vi "ContextHelpEditor VI.vi"(5 "Shift Pressed?":bool, 6 "ComboBox Text":string, 7 "Executed on Frontpanel?":bool, 8 "error in (no error)":errorcluster, 11 "VI Ref":refnum<vi>) -> (0 "error out":errorcluster)   [LabVIEW 2020, in "ContextHelpEditor.lvlib"]
uses:
  ContextHelpEditor.lvlib
  Data--cluster.ctl
  ControlRef--cluster.ctl
  <vilib>/picture/picture.llb/imagedata.ctl
  TabbedControl--cluster.ctl
  <vilib>/Platform/browser.llb/Open URL in Default Browser (string).vi
panel:
  in  "Controls":i32(listbox)
  in  "Help":bool
  in  "Delete VI Title":bool
  in  "VI Title":string caption="Title"
  in  "Description":string
  # "Use <b> and </b> tags around any text in the description you want to format as bold. \n\nUse TAB (forward) and SHIFT+TAB (backward) to jump between entries. \nESC will close the editor and change the VI properties. The VI won't be saved automatically."
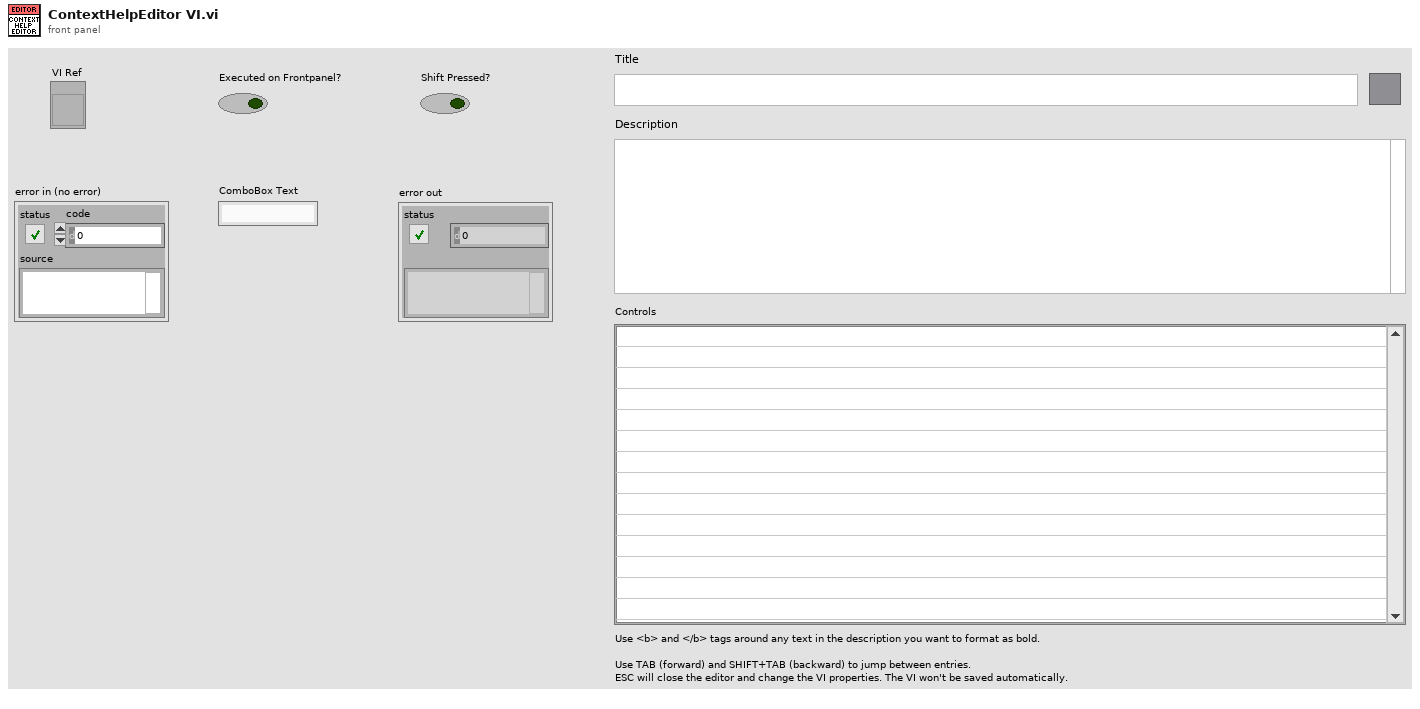
[diagram p1: front panel]
types:
  T1 = enum32{"Invalid", "Standard", "Closed", "Hidden", "Minimized", "Maximized"}
  T2 = enum32{"invalid app kind", "Development System", "Run Time System", "Student Edition", "Embedded LabVIEW", "Evaluation", "Custom"}
  T3 = typedef "ContextHelpEditor.lvlib/Data--cluster.ctl" = cluster{"Core":cluster{"Current VI Reference":refnum<vi>, "Close Panel on Exit?":bool}, "Controls":T4[], "QuickDrop":cluster{"VI Ref":refnum<vi>, "Executed on Frontpanel?":bool, "Shift Pressed?":bool, "ComboBox Text":string}, "TabbedControls":T6[]}
  T4 = typedef "ContextHelpEditor.lvlib/ControlRef--cluster.ctl" = cluster{"Ref":refnum<vi>, "Label":string, "Description":string, "Image":T5}
  T5 = typedef "imagedata.ctl" = cluster{"image type":i32, "image depth":i32, "image":u8[], "mask":u8[], "colors":u32[], "Rectangle":cluster{"left":i16, "top":i16, "right":i16, "bottom":i16}}
  T6 = typedef "ContextHelpEditor.lvlib/TabbedControl--cluster.ctl" = cluster{"Label":string, "Control Ref":refnum<vi>, "ClassName":string}
  T7 = enum32{"invalid VI type", "Standard VI", "Control VI", "Global VI", "Polymorphic VI", "Configuration VI", "SubSystem", "Facade VI", "Method VI", "Statechart Diagram VI"}
  T8 = typedef "eventvkey.ctl" = enum16{"ASCII", "Enter", "Return", "Shift", "Ctrl", "Alt", "Cmd", "Opt", "Caps", "NumLock", "Clear", "Break", "Up", "Down", "Left", "Right", "Insert", "Delete", "Home", "End", "PageUp", "PageDown", "Escape", "Help", "Pause", "ScrollLock", "F1", "F2", "F3", "F4", "F5", "F6", "F7", "F8", "F9", "F10", "F11", "F12", "F13", "F14", "F15", "F16", "F17", "F18", "F19", "F20", "F21", "F22", "F23", "F24", "Play", "VolumeUp", "VolumeDown", "Mute", "Two Byte Char"}
  T9 = cluster{"Shift":bool, "Ctrl":bool, "Alt":bool, "Cmd":bool, "Opt":bool}
  T10 = typedef "LVPoint32TypeDef.ctl" = cluster{"Horizontal":i32, "Vertical":i32}
  T11 = typedef "LVRowAndColumnTypeDef.ctl" = cluster{"Row":i32, "Column":i32}
  T12 = cluster{"Current VI Reference":refnum<vi>, "Close Panel on Exit?":bool}
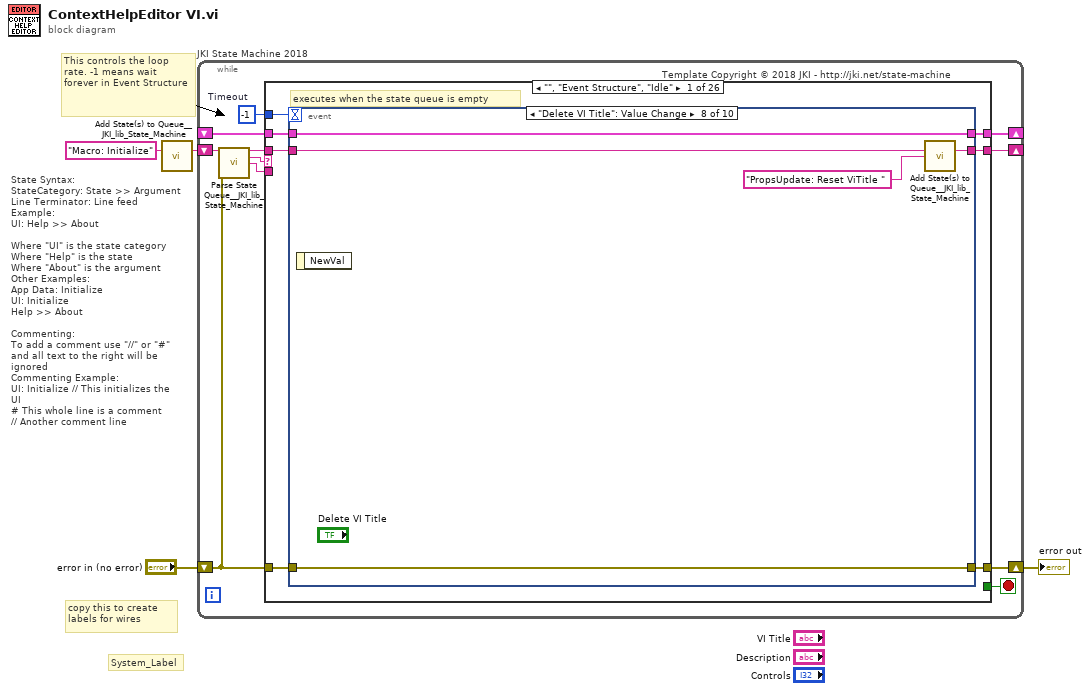
[diagram p0: block diagram]
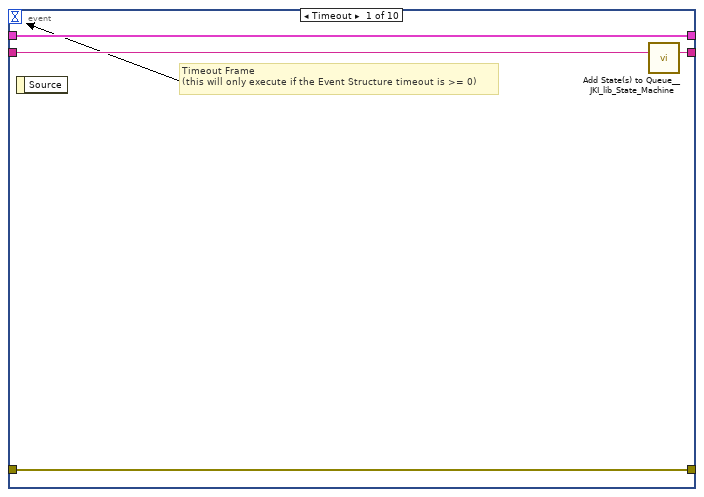
[diagram p2: hidden frame]
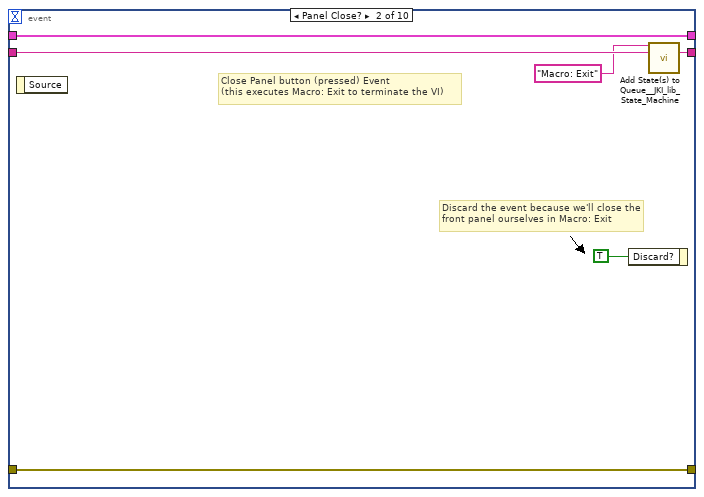
[diagram p3: hidden frame]
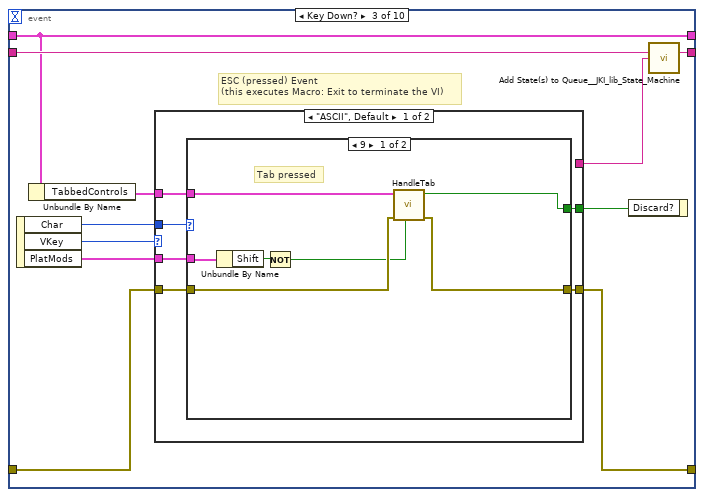
[diagram p4: hidden frame]
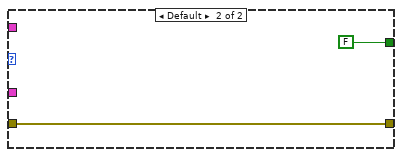
[diagram p5: hidden frame]
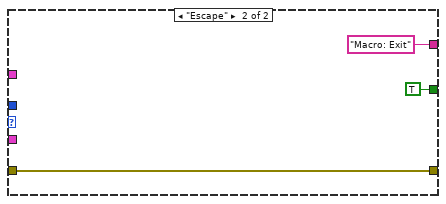
[diagram p6: hidden frame]
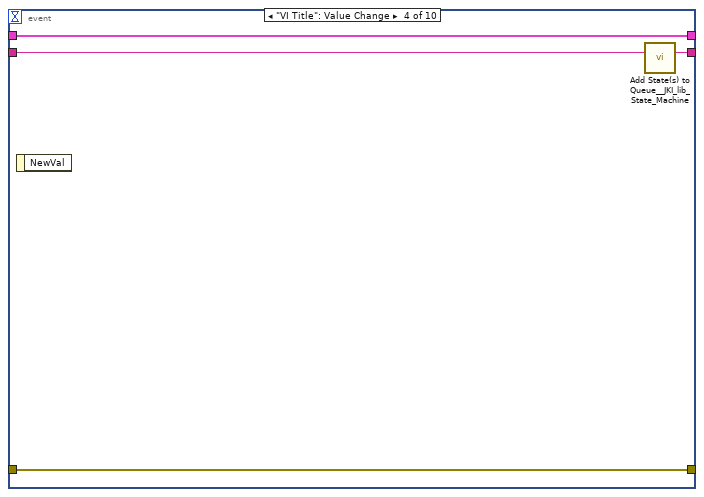
[diagram p7: hidden frame]
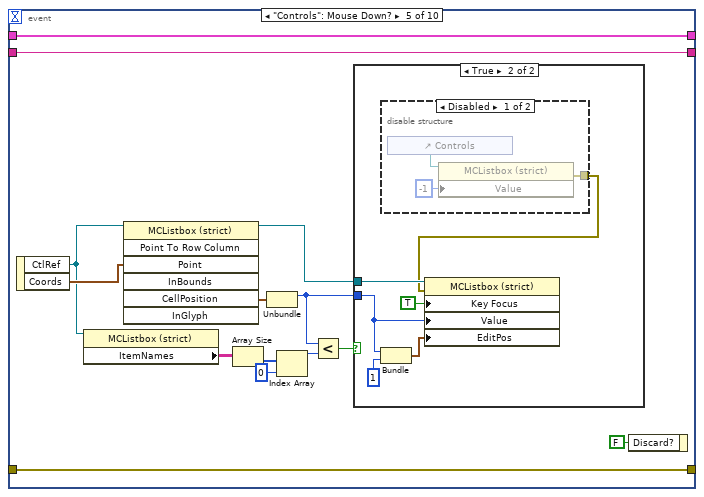
[diagram p8: hidden frame]
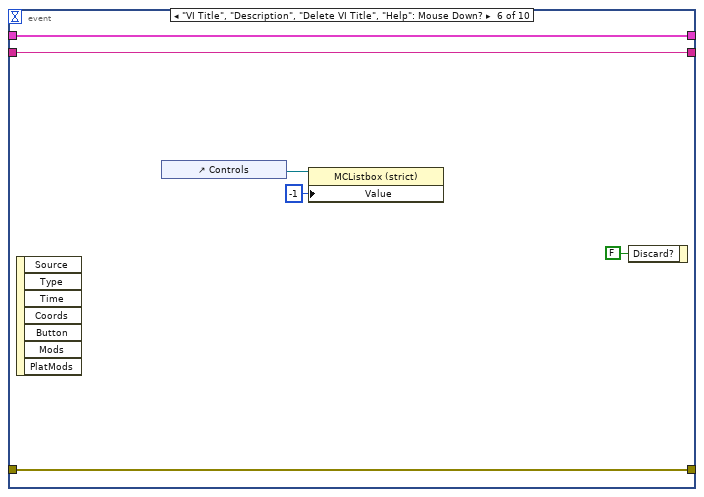
[diagram p11: hidden frame]
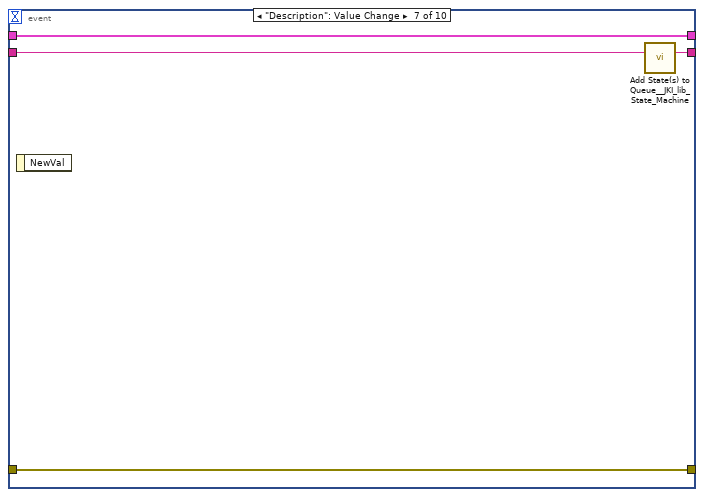
[diagram p12: hidden frame]
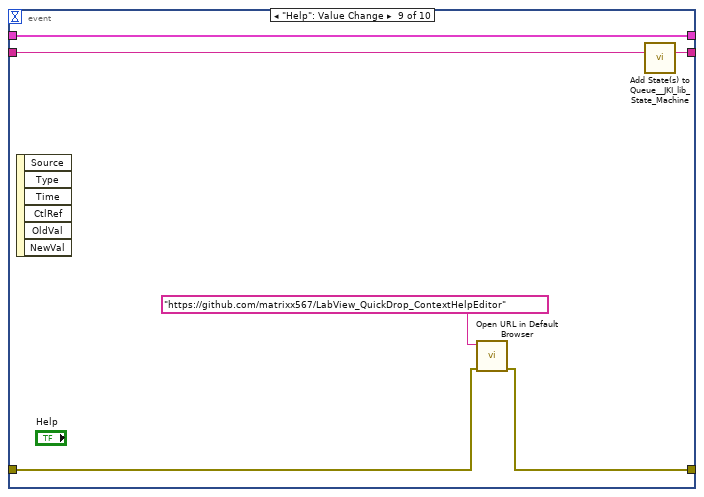
[diagram p13: hidden frame]
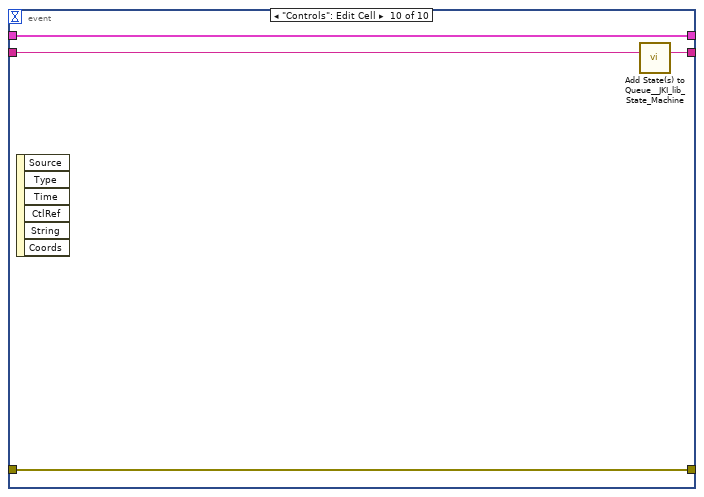
[diagram p14: hidden frame]
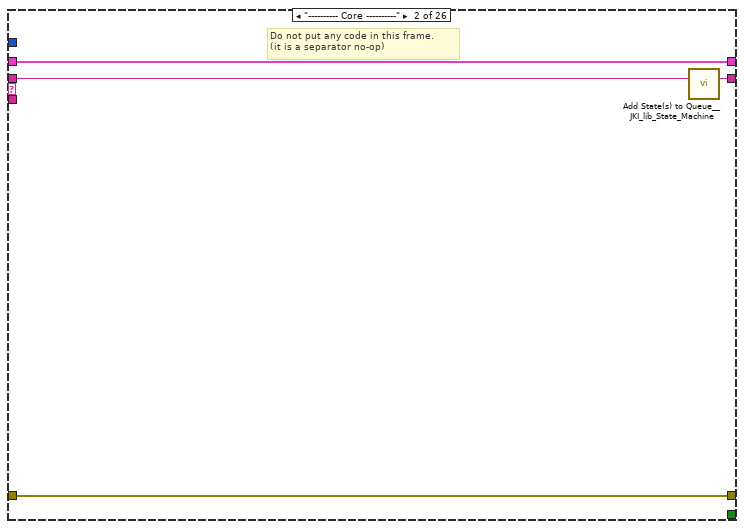
[diagram p15: hidden frame]
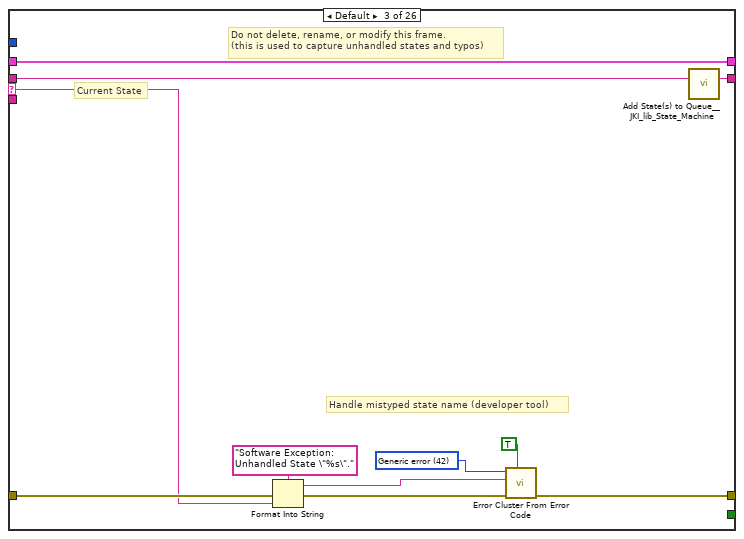
[diagram p16: hidden frame]
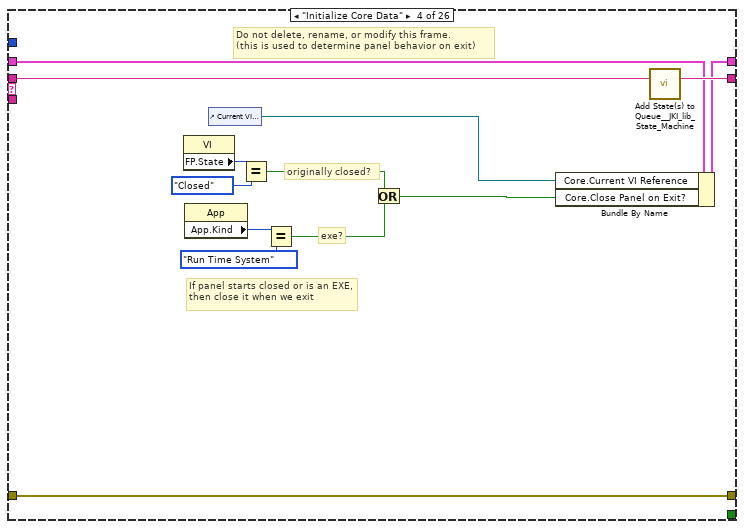
[diagram p17: hidden frame]
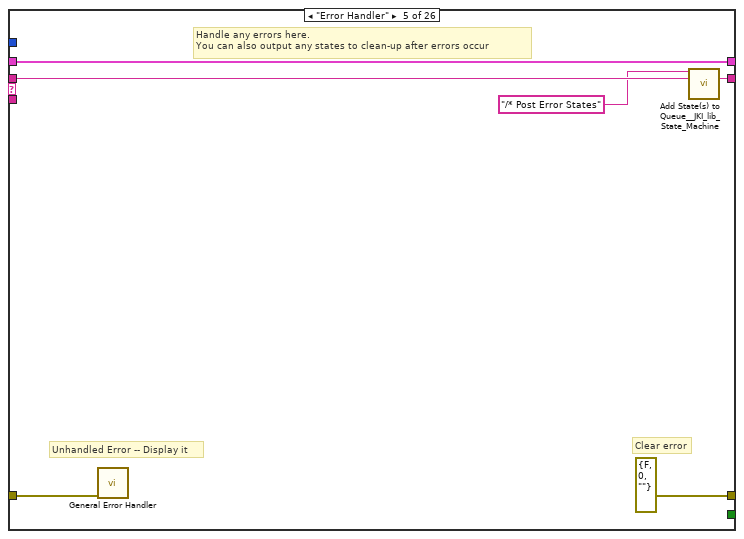
[diagram p18: hidden frame]
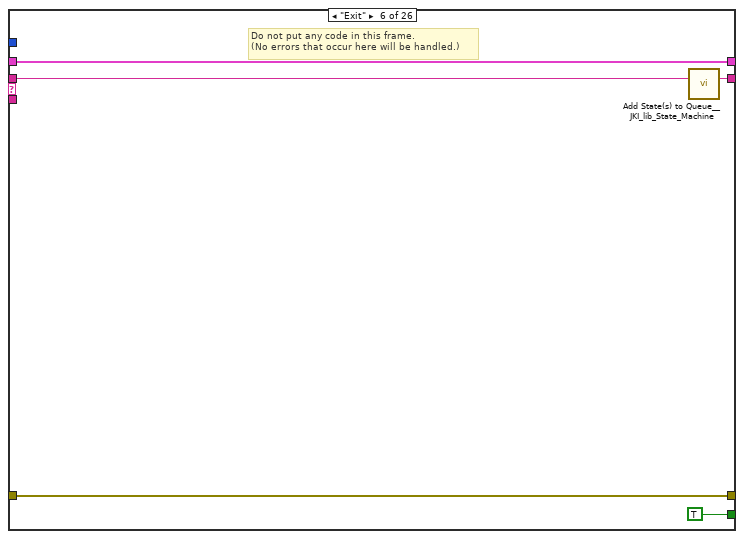
[diagram p19: hidden frame]
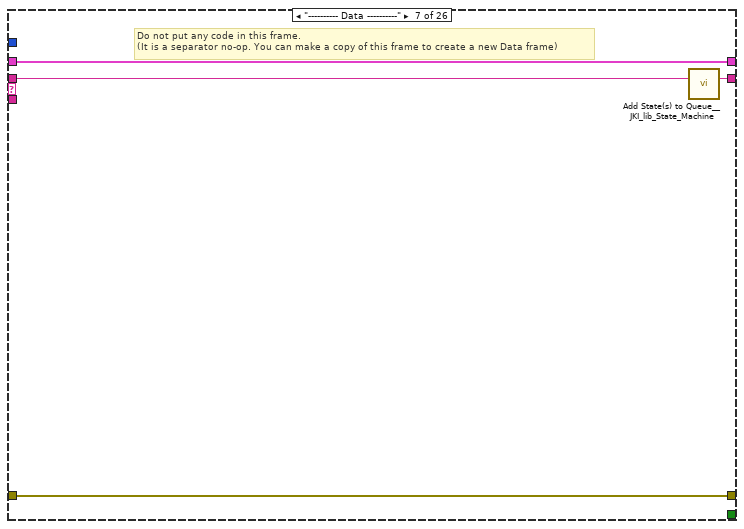
[diagram p20: hidden frame]
diagram:
  # "State Syntax:\nStateCategory: State >> Argument\nLine Terminator: Line feed\nExample:\nUI: Help >> About\n\nWhere \"UI\" is the state category\nWhere \"Help\" is the state\nWhere \"About\" is the argument\nOther Examples:\nApp Data: Initialize\nUI: Initialize\nHelp >> About\n\nCommenting:\nTo add a comment use \"//\" or \"#\" and all text to the right will be ignored\nCommenting Example:\nUI: Initialize // This initializes the UI\n# This whole line is a comment\n// Another comment line"
  # "copy this to create labels for wires"
  # "This controls the loop rate. -1 means wait forever in Event Structure"
  # "System_Label"
  n1 = call <vilib>:"Add State(s) to Queue__JKI_lib_State_Machine.vi"("State(s) in (\"\")"="Macro: Initialize") -> ("States Out"=w4:string)  [unwired: 14 in]
  n2 = while "JKI State Machine 2018" {
    shift-right: [w8] -> _
    shift-left: _ -> [w7]
    shift-right: [w11] -> w1
    shift-left: "error in (no error)" -> [w5]
    shift-right: [w10] -> _
    shift-left: w4 -> [w12]
    stop <- w9 stop-if-true
    w6 = -1  # Timeout
    # "Template Copyright © 2018 JKI - http://jki.net/state-machine"
    n3 = call <vilib>:"Parse State Queue__JKI_lib_State_Machine.vi"("State Queue"=w12, "Error In (no error)"=w5) -> ("Remaining States"=w14:string, "Current State"=w15:string, "Arguments"=w13:string)  [unwired: 11 in]
    n4 = case shown="\"\", \"Event Structure\", \"Idle\"" w15 {
      selector: w15 -> [_ _ w118 _ _ _ _ _ _ _ _ _ _ _ _ _ _ _ _ _ _ _ _ _ _ _]
      tunnel: w14 -> [w22 w117 w122 w141 w147 w152 w156 w167 w177 w194 w198 w210 w216 w227 w302 w314 w335 w354 w363 w368 w380 w384 w394 w406 w444 w478]
      tunnel: w13 -> [_ _ _ _ _ _ _ _ _ _ _ _ w211 w221 _ _ _ _ _ _ _ _ _ _ _ _]
      tunnel: w7 -> [w20 w114 w120 w134 w144 w150 w153 _ w174 w191 w195 w202 w214 w223 w295 w312 w333 w352 w360 w364 w377 w381 w391 w404 w442 w476]
      tunnel: [w19 w115 w124 w138 errorcluster {"status"=FALSE, "code"=0, "source"=""} ("error out") w149 w154 w162 w168 w190 w196 w201 w212 w224 w296 w310 w331 w351 w361 w366 w378 w382 w389 w396 w434 w473] -> w11
      tunnel: w5 -> [w18 w115 w123 w138 w143 w149 w154 w164 w170 w190 w196 w201 w213 w225 _ w309 _ _ w361 w366 w378 w382 w388 w395 w433 w472]
      tunnel: [w21 w116 w121 w140 w146 w151 w155 w166 w176 w193 w197 w209 w215 w226 w301 w313 w334 w353 w362 w367 w379 w383 w393 w405 w443 w477] -> w10
      tunnel: [_ _ _ _ _ TRUE _ _ _ _ _ _ _ _ _ _ _ _ _ _ _ _ _ _ _ _] -> w9
      tunnel: [w17 w114 w120 w139 w144 w150 w153 w165 w175 w191 w195 w202 w214 w223 w300 w312 w333 w352 w360 w364 w377 w381 w391 w404 w442 w476] -> w8
      tunnel: w6 -> [w16 _ _ _ _ _ _ _ _ _ _ _ _ _ _ _ _ _ _ _ _ _ _ _ _ _]
      frame "", "Event Structure", "Idle" {
        # "executes when the state queue is empty"
        n5 = event shown="[7] \"Delete VI Title\": Value Change" {
          selector: _ -> [_ _ _ _ _ _ _ _ _ _]
          dyn-events: _ -> [_ _ _ _ _ _ _ _ _ _]
          timeout: w16 -> [_ _ _ _ _ _ _ _ _ _]
          tunnel: w22 -> [w26 w32 w43 w64 w79 w94 w97 w102 w108 w112]
          tunnel: [w25 w31 w42 w65 w79 w94 w98 w103 w109 w111] -> w21
          tunnel: w20 -> [w23 w29 w36 w63 w77 w92 w96 w101 w107 w113]
          tunnel: [w24 w30 w37 w62 w78 w93 w95 w99 w104 w110] -> w19
          tunnel: w18 -> [w24 w30 w38 w62 w78 w93 w95 w99 w105 w110]
          tunnel: [w23 w29 w36 w63 w77 w92 w96 w101 w107 w113] -> w17
          event Timeout {
            # "Timeout Frame\n(this will only execute if the Event Structure timeout is >= 0)"
            n6 = event-data() -> ()  [unwired: 1 in, 1 out]
            n7 = call <vilib>:"Add State(s) to Queue__JKI_lib_State_Machine.vi"("State(s) in (\"\")"=w26) -> ("States Out"=w25:string)  [unwired: 14 in]
          }
          event Panel Close? {
            # "Discard the event because we'll close the front panel ourselves in Macro: Exit"
            # "Close Panel button (pressed) Event\n(this executes Macro: Exit to terminate the VI)"
            n8 = event-data() -> ()  [unwired: 1 in, 1 out]
            n9 = event-data("Discard?"=TRUE) -> ()  [unwired: 1 in, 1 out]
            n10 = call <vilib>:"Add State(s) to Queue__JKI_lib_State_Machine.vi"("State(s) in Front (\"\")"="Macro: Exit", "State(s) in (\"\")"=w32) -> ("States Out"=w31:string)  [unwired: 13 in]
          }
          event Key Down? {
            # "ESC (pressed) Event\n(this executes Macro: Exit to terminate the VI)"
            n11 = event-data() -> ("Char"=w39:i16, "VKey"=w41:T8, "PlatMods"=w34:T9)  [unwired: 1 in]
            n12 = Unbundle By Name(w36) -> ("TabbedControls"=w35:T6[])
            n13 = case shown="\"ASCII\", Default" w41 {
              tunnel: [_ "Macro: Exit"] -> w33
              tunnel: [w48 TRUE] -> w40
              tunnel: w39 -> [w49 _]
              tunnel: [w47 w61] -> w37
              tunnel: w38 -> [w46 w61]
              tunnel: w35 -> [w45 _]
              tunnel: w34 -> [w44 _]
              frame "ASCII", Default {
                n14 = case shown="9" w49 {
                  tunnel: [w56 FALSE] -> w48
                  tunnel: [w54 w57] -> w47
                  tunnel: w46 -> [w55 w57]
                  tunnel: w45 -> [w53 _]
                  tunnel: w44 -> [w52 _]
                  frame 9 {
                    # "Tab pressed"
                    n15 = Unbundle By Name(w52) -> ("Shift"=w51:bool)
                    n16 = Not(x=w51) -> (.not. x?=w50:bool)
                    n17 = call "HandleTab.vi"("Forward?"=w50, "error in (no error)"=w55, "TabbedControls"=w53) -> ("error out"=w54:errorcluster, "Discard?"=w56:bool)  [unwired: 7 in]
                  }
                  frame Default {
                  }
                }
              }
              frame "Escape" {
              }
            }
            n18 = event-data("Discard?"=w40) -> ()  [unwired: 1 in, 1 out]
            n19 = call <vilib>:"Add State(s) to Queue__JKI_lib_State_Machine.vi"("State(s) in (\"\")"=w43, "State(s) at Back (\"\")"=w33) -> ("States Out"=w42:string)  [unwired: 13 in]
          }
          event "VI Title": Value Change {
            n20 = event-data() -> ()  [unwired: 1 in, 1 out]
            n21 = call <vilib>:"Add State(s) to Queue__JKI_lib_State_Machine.vi"("State(s) in (\"\")"=w64) -> ("States Out"=w65:string)  [unwired: 14 in]
          }
          event "Controls": Mouse Down? {
            n22 = event-data() -> ("CtlRef"=w72:refnum<vi>, "Coords"=w76:T10)  [unwired: 1 in]
            n23 = property class="MCListbox (strict)"(reference=w72) -> ("ItemNames"=w71:string[][])  [unwired: 1 in, 2 out]
            n24 = invoke class="MCListbox (strict)" method="Point To Row Column"(reference=w72, "Point"=w76) -> (reference out=w75:refnum<vi>, "CellPosition"=w74:T11)  [unwired: 5 in, 5 out]
            n25 = Array Size(array=w71) -> (size(s)=w67:i32[])
            n26 = Unbundle(w74) -> ("Row"=w70:i32)  [unwired: 1 out]
            n27 = Index Array(array=w67, index=0) -> (element=w66:i32)
            n28 = Less?(x=w70, y=w66) -> (x < y?=w69:bool)
            n29 = case shown="True" w69 {
              tunnel: w75 -> [_ w83]
              tunnel: w70 -> [_ w80]
              frame False {
                # "ignore empty lines"
              }
              frame True {
                n30 = Bundle("Row"=w80, "Row"=1) -> (w85:cluster{"Row":i32, "Row":i32})  [unwired: 1 in]
                n31 = disable-structure shown="Disabled" {
                  disable-tunnel: [w87 _] -> w81
                  frame Disabled {
                    n32 = control-ref of="Controls"() -> (w88:refnum<vi>)
                    n33 = property class="MCListbox (strict)"(reference=w88, "Value"=-1) -> (error out=w87:errorcluster)  [unwired: 1 in, 1 out]
                  }
                  frame Enabled {
                  }
                }
                n34 = property class="MCListbox (strict)"(reference=w83, error in=w81, "Key Focus"=TRUE, "Value"=w80, "EditPos"=w85) -> ()  [unwired: 2 out]
              }
            }
            n35 = event-data("Discard?"=FALSE) -> ()  [unwired: 1 in, 1 out]
          }
          event "VI Title", "Description", "Delete VI Title", "Help": Mouse Down? {
            n36 = event-data() -> ()  [unwired: 1 in, 7 out]
            n37 = control-ref of="Controls"() -> (w90:refnum<vi>)
            n38 = property class="MCListbox (strict)"(reference=w90, "Value"=-1) -> ()  [unwired: 1 in, 2 out]
            n39 = event-data("Discard?"=FALSE) -> ()  [unwired: 1 in, 1 out]
          }
          event "Description": Value Change {
            n40 = event-data() -> ()  [unwired: 1 in, 1 out]
            n41 = call <vilib>:"Add State(s) to Queue__JKI_lib_State_Machine.vi"("State(s) in (\"\")"=w97) -> ("States Out"=w98:string)  [unwired: 14 in]
          }
          event "Delete VI Title": Value Change {
            n42 = event-data() -> ()  [unwired: 1 in, 1 out]
            n43 = call <vilib>:"Add State(s) to Queue__JKI_lib_State_Machine.vi"("State(s) in (\"\")"=w102, "State(s) at Back (\"\")"="PropsUpdate: Reset ViTitle ") -> ("States Out"=w103:string)  [unwired: 13 in]
          }
          event "Help": Value Change {
            n44 = event-data() -> ()  [unwired: 1 in, 6 out]
            n45 = call-poly <vilib>:"Open URL in Default Browser.vi"("error in (no error)"=w105, "URL"="https://github.com/matrixx567/LabView_QuickDrop_ContextHelpEditor") -> ("error out"=w104:errorcluster)  [unwired: 4 in, 1 out]
            n46 = call <vilib>:"Add State(s) to Queue__JKI_lib_State_Machine.vi"("State(s) in (\"\")"=w108) -> ("States Out"=w109:string)  [unwired: 14 in]
          }
          event "Controls": Edit Cell {
            n47 = event-data() -> ()  [unwired: 1 in, 6 out]
            n48 = call <vilib>:"Add State(s) to Queue__JKI_lib_State_Machine.vi"("State(s) in (\"\")"=w112) -> ("States Out"=w111:string)  [unwired: 14 in]
          }
        }
      }
      frame "---------- Core ----------" {
        # "Do not put any code in this frame.\n(it is a separator no-op)"
        n49 = call <vilib>:"Add State(s) to Queue__JKI_lib_State_Machine.vi"("State(s) in (\"\")"=w117) -> ("States Out"=w116:string)  [unwired: 14 in]
      }
      frame Default {
        w127 = 42 items=["No error", "Argument error", "Memory is full", "Out of zone", "End of file", "File already open", "Generic file I/O error", "File not found", "File permission error", "Disk is full", "Duplicate path", "Too many files open", "System feature not enabled", "Resource file not found", "Cannot add resource", "Resource not found", "Image not found", "Image memory error", "Pen does not exist", "Config type invalid", "Config token not found", "Config parse error", "Config memory error", "Bad external code format", "Bad external code offset", "External code not present", "Null window", "Destroy window error", "Null menu", "Print aborted", "Bad print record", "Print driver error", "Windows error during printing", "Memory error during printing", "Print dialog error", "Generic print error", "Invalid device refnum", "Device not found", "Device parameter error", "Device unit error", "Cannot open device", "Device call aborted", "Generic error", "Cancelled by user", "Object ID too low", "Object ID too high", "Object not in heap", "Unknown heap", "Unknown object (invalid DefProc)", "Unknown object (DefProc not in table)", "Message out of range", "Invalid (null) method", "Unknown message", "Manager call not supported", "Bad address", "Network operation in progress", "Network operation timed out", "Connection is busy", "Network attribute not supported", "Network error", "Address in use", "System out of memory", "Connection aborted", "Connection refused", "Not connected", "Already connected", "Connection closed", "Initialization error (interapplication manager)", "Bad occurrence", "Wait on unbound occurrence handler", "Occurrence queue overflow", "Datalog type conflict", "Unused", "Unrecognized type (interapplication manager)", "Memory corrupt", "Failed to make temporary DLL", "Old CIN version", "Drag socket not found", "Failed to load drop-object", "Failed to register OLE object", "Failed to release OLE object", "Format specifier type mismatch", "Unknown format specifier", "Too few format specifiers", "Too many format specifiers", "Scan failed", "Newer CIN version", "Error converting to variant", "Runtime menu error", "Password tampered", "Variant attribute not found", "Incompatible variant data type", "Event data is not available", "Event Store is not present", "Occurrence is not found", "Event Queue is not created", "Event info is not available", "Refnum passed is NULL", "Error retrieving Class GUID", "Error retrieving CoClass GUID", "Error retrieving TypeLib GUID.", "Bad built application magic bytes.", "Specific driver is different from the specific driver associated with the Logical Name.", "There is no session opened to the class driver.", "Max Error", "MAX - Error with config objects", "MAX - Error loading configuration", "MAX - Group not supported"]
        # "Current State"
        # "Do not delete, rename, or modify this frame.\n(this is used to capture unhandled states and typos)"
        # "Handle mistyped state name (developer tool)"
        n50 = Format Into String(format string="Software Exception: Unhandled State \"%s\"." ("message"), error in=w123, w118) -> (resulting string=w126:string, error out=w125:errorcluster)  [unwired: 1 in]
        n51 = call <vilib>:"Error Cluster From Error Code.vi"("show call chain? (False)"=TRUE, "error in (no error)"=w125, "error message (\"\")"=w126, "error code (0)"=w127) -> ("error out"=w124:errorcluster)  [unwired: 5 in]
        n52 = call <vilib>:"Add State(s) to Queue__JKI_lib_State_Machine.vi"("State(s) in (\"\")"=w122) -> ("States Out"=w121:string)  [unwired: 14 in]
      }
      frame "Initialize Core Data" {
        # "Do not delete, rename, or modify this frame.\n(this is used to determine panel behavior on exit)"
        # "originally closed?"
        # "exe?"
        # "If panel starts closed or is an EXE, then close it when we exit"
        n53 = property class="VI"() -> ("FP.State"=w131:T1)  [unwired: 2 in, 2 out]
        n54 = property class="App"() -> ("App.Kind"=w137:T2)  [unwired: 2 in, 2 out]
        n55 = control-ref of="Current VI Reference"() -> (w132:refnum<vi>)
        n56 = Equal?(x=w131, y=T1."Closed" ("Front Panel Window:State")) -> (x = y?=w129:bool)
        n57 = Equal?(x=w137, y=T2."Run Time System" ("Application:Kind")) -> (x = y?=w135:bool)
        n58 = Or(x=w129, y=w135) -> (x .or. y?=w133:bool)
        n59 = Bundle By Name(cluster=w134, "Core.Current VI Reference"=w132, "Core.Close Panel on Exit?"=w133) -> (w139:T3)
        n60 = call <vilib>:"Add State(s) to Queue__JKI_lib_State_Machine.vi"("State(s) in (\"\")"=w141) -> ("States Out"=w140:string)  [unwired: 14 in]
      }
      frame "Error Handler" {
        # "Unhandled Error -- Display it"
        # "Handle any errors here.\nYou can also output any states to clean-up after errors occur"
        # "Clear error"
        n61 = call <vilib>:"General Error Handler.vi"("error in (no error)"=w143) -> ()  [unwired: 10 in, 5 out]
        n62 = call <vilib>:"Add State(s) to Queue__JKI_lib_State_Machine.vi"("State(s) in Front (\"\")"="/* Post Error States", "State(s) in (\"\")"=w147) -> ("States Out"=w146:string)  [unwired: 13 in]
      }
      frame "Exit" {
        # "Do not put any code in this frame.\n(No errors that occur here will be handled.)"
        n63 = call <vilib>:"Add State(s) to Queue__JKI_lib_State_Machine.vi"("State(s) in (\"\")"=w152) -> ("States Out"=w151:string)  [unwired: 14 in]
      }
      frame "---------- Data ----------" {
        # "Do not put any code in this frame.\n(It is a separator no-op. You can make a copy of this frame to create a new Data frame)"
        n64 = call <vilib>:"Add State(s) to Queue__JKI_lib_State_Machine.vi"("State(s) in (\"\")"=w156) -> ("States Out"=w155:string)  [unwired: 14 in]
      }
      frame "Data: Initialize" {
        w163 = T12 {"Current VI Reference"=refnum, "Close Panel on Exit?"=FALSE}  # Core
        # "do not delete - used by framework"
        # "Data names and types of shift register data are defined by this bundle."
        # "Initialize the shift-register data, here.\n(data names are defined by what you wire into the bundle function)"
        n65 = Merge Errors(w164) -> (w162:errorcluster)
        n66 = Bundle By Name(cluster=T3 {"Core"={"Current VI Reference"=refnum, "Close Panel on Exit?"=FALSE}, "Controls"=[], "QuickDrop"={"VI Ref"=refnum, "Executed on Frontpanel?"=FALSE, "Shift Pressed?"=FALSE, "ComboBox Text"=""}, "TabbedControls"=[]}, "Core"=w163, "QuickDrop.VI Ref"="VI Ref", "QuickDrop.Executed on Frontpanel?"="Executed on Frontpanel?", "QuickDrop.ComboBox Text"="ComboBox Text", "QuickDrop.Shift Pressed?"="Shift Pressed?") -> (w165:T3)
        n67 = call <vilib>:"Add State(s) to Queue__JKI_lib_State_Machine.vi"("State(s) in (\"\")"=w167) -> ("States Out"=w166:string)  [unwired: 14 in]
      }
      frame "Data: LoadControlFromVI" {
        # "Initialize the shift-register data, here.\n(data names are defined by what you wire into the bundle function)"
        n68 = Unbundle By Name(w174) -> ("QuickDrop.VI Ref"=w172:refnum<vi>)
        n69 = property class="VI"(reference=w172) -> ("VIType"=w171:T7)  [unwired: 1 in, 2 out]
        n70 = case shown="\"Control VI\"" w171 {
          tunnel: w172 -> [_ w181 w189]
          tunnel: [_ w180 w187] -> w173
          tunnel: [_ w178 w188] -> w169
          frame Default {
          }
          frame "Standard VI" {
            w182 = FALSE  # LoadAllControls
            n71 = call "ExtractControlRefsFromVi.vi"("ShowAllControls?"=w182, "VI in"=w181) -> ("error out"=w186:errorcluster, "Controls"=w183:T4[])  [unwired: 8 in]
            n72 = call "ExtractControlRefsFromVi.vi"("Indicators"=TRUE, "ShowAllControls?"=w182, "VI in"=w181) -> ("error out"=w185:errorcluster, "Controls"=w179:T4[])  [unwired: 7 in]
            n73 = Merge Errors(w186, w185) -> (w178:errorcluster)
            n74 = Build Array (concatenate)(w183, w179) -> (w180:T4[])
          }
          frame "Control VI" {
            n75 = call "ExtractControlRefsFromTypedef.vi"("VI in"=w189) -> ("error out"=w188:errorcluster, "Controls"=w187:T4[])  [unwired: 9 in]
          }
        }
        n76 = Bundle By Name(cluster=w174, "Controls"=w173) -> (w175:T3)
        n77 = Merge Errors(w170, w169) -> (w168:errorcluster)
        n78 = call <vilib>:"Add State(s) to Queue__JKI_lib_State_Machine.vi"("State(s) in (\"\")"=w177) -> ("States Out"=w176:string)  [unwired: 14 in]
      }
      frame "Data: Cleanup" {
        # "Cleanup any data and references, here.\n(this is called automatically, by the Macro: Exit)"
        n79 = Unbundle By Name(w191) -> ("Core.Current VI Reference"=w192:refnum<vi>)
        n80 = Close Reference(reference=w192) -> ()  [unwired: 1 in, 1 out]
        n81 = call <vilib>:"Add State(s) to Queue__JKI_lib_State_Machine.vi"("State(s) in (\"\")"=w194) -> ("States Out"=w193:string)  [unwired: 14 in]
      }
      frame "---------- UI ----------" {
        # "Do not put any code in this frame.\n(It is a separator no-op. You can make a copy of this frame to create a new UI frame)"
        n82 = call <vilib>:"Add State(s) to Queue__JKI_lib_State_Machine.vi"("State(s) in (\"\")"=w198) -> ("States Out"=w197:string)  [unwired: 14 in]
      }
      frame "UI: Initialize" {
        # "Initialize the User Interface, here.\n(this is called automatically, by the Macro: Init)"
        n83 = Unbundle By Name(w202) -> ("Core.Current VI Reference"=w207:refnum<vi>)
        n84 = Unbundle By Name(w202) -> ("QuickDrop.VI Ref"=w204:refnum<vi>)
        n85 = property class="VI"(reference=w204) -> ("Front Panel.Title"=w203:string)  [unwired: 1 in, 2 out]
        n86 = control-ref of="Controls"() -> (w208:refnum<vi>)
        n87 = Concatenate Strings("ContextHelpEditor - " ("string"), w203) -> (w206:string)
        n88 = property class="VI"(reference=w207, "Front Panel.Title"=w206) -> ()  [unwired: 1 in, 2 out]
        n89 = property class="MCListbox (strict)"(reference=w208, "SelColor"=u32 13816530, "Value"=-1) -> ()  [unwired: 1 in, 2 out]
        n90 = call <vilib>:"Add State(s) to Queue__JKI_lib_State_Machine.vi"("State(s) in (\"\")"=w210) -> ("States Out"=w209:string)  [unwired: 14 in]
      }
      frame "UI: Cursor Set" {
        # "Argument"
        # "Set and Unset Cursor Busy.\n(Usage: \"UI: Cursor Set >> Busy|Idle\")"
        n91 = case shown="\"Busy\"" w211 {
          tunnel: w213 -> [w218 w220]
          tunnel: [w217 w219] -> w212
          frame "Idle", Default {
            n92 = call <vilib>:"Unset Busy.vi"("error in (no error)"=w218) -> ("error out"=w217:errorcluster)  [unwired: 10 in]
          }
          frame "Busy" {
            n93 = call <vilib>:"Set Busy.vi"("error in (no error)"=w220) -> ("error out"=w219:errorcluster)  [unwired: 9 in, 1 out]
          }
        }
        n94 = call <vilib>:"Add State(s) to Queue__JKI_lib_State_Machine.vi"("State(s) in (\"\")"=w216) -> ("States Out"=w215:string)  [unwired: 14 in]
      }
      frame "UI: Front Panel State" {
        # "Argument"
        # "Set Front Panel Open or Closed\n(Usage: \"UI: Front Panel State >> Open|Close\")"
        n95 = Unbundle By Name(w223) -> ("Core.Current VI Reference"=w222:refnum<vi>)
        n96 = case shown="\"Open\", \"Standard\", Default" w221 {
          tunnel: w225 -> [w233 w248 w259 w272 w285]
          tunnel: [w235 w249 w261 w274 w287] -> w224
          tunnel: w222 -> [w234 w246 w260 w273 w286]
          frame "Open", "Standard", Default {
            w228 = T1."Standard" ("State")
            n97 = property class="VI"(reference=w234, error in=w233) -> (reference out=w231:refnum<vi>, error out=w232:errorcluster, "FP.State"=w230:T1)
            n98 = Not Equal?(x=w230, y=w228) -> (x != y?=w229:bool)
            n99 = case shown="True" w229 {
              tunnel: [w239 w241] -> w235
              tunnel: w232 -> [w238 w241]
              tunnel: w231 -> [w237 _]
              tunnel: w228 -> [w236 _]
              frame True {
                n100 = invoke class="VI" method="FP.Open"(reference=w237, error in=w238, "Activate"=TRUE, "State"=w236) -> (error out=w239:errorcluster)  [unwired: 1 in, 4 out]
              }
              frame False {
              }
            }
          }
          frame "Close", "Closed" {
            n101 = property class="VI"(reference=w246, error in=w248) -> (reference out=w245:refnum<vi>, error out=w247:errorcluster, "FP.State"=w243:T1)
            n102 = Not Equal?(x=w243, y=T1."Closed" ("Front Panel Window:State")) -> (x != y?=w242:bool)
            n103 = case shown="True" w242 {
              tunnel: [w250 w253] -> w249
              tunnel: w247 -> [w250 w252]
              tunnel: w245 -> [_ w251]
              frame False {
              }
              frame True {
                n104 = invoke class="VI" method="FP.Close"(reference=w251, error in=w252) -> (error out=w253:errorcluster)  [unwired: 1 in, 2 out]
              }
            }
          }
          frame "Hidden", "Hide" {
            w254 = T1."Hidden" ("State")
            n105 = property class="VI"(reference=w260, error in=w259) -> (reference out=w257:refnum<vi>, error out=w258:errorcluster, "FP.State"=w256:T1)
            n106 = Not Equal?(x=w256, y=w254) -> (x != y?=w255:bool)
            n107 = case shown="True" w255 {
              tunnel: [w265 w266] -> w261
              tunnel: w258 -> [w264 w266]
              tunnel: w257 -> [w263 _]
              tunnel: w254 -> [w262 _]
              frame True {
                n108 = invoke class="VI" method="FP.Open"(reference=w263, error in=w264, "State"=w262) -> (error out=w265:errorcluster)  [unwired: 2 in, 4 out]
              }
              frame False {
              }
            }
          }
          frame "Minimize", "Minimized" {
            w267 = T1."Minimized" ("State")
            n109 = property class="VI"(reference=w273, error in=w272) -> (reference out=w270:refnum<vi>, error out=w271:errorcluster, "FP.State"=w269:T1)
            n110 = Not Equal?(x=w269, y=w267) -> (x != y?=w268:bool)
            n111 = case shown="True" w268 {
              tunnel: [w278 w279] -> w274
              tunnel: w271 -> [w277 w279]
              tunnel: w270 -> [w276 _]
              tunnel: w267 -> [w275 _]
              frame True {
                n112 = invoke class="VI" method="FP.Open"(reference=w276, error in=w277, "State"=w275) -> (error out=w278:errorcluster)  [unwired: 2 in, 4 out]
              }
              frame False {
              }
            }
          }
          frame "Maximize", "Maximized" {
            w280 = T1."Maximized" ("State")
            n113 = property class="VI"(reference=w286, error in=w285) -> (reference out=w283:refnum<vi>, error out=w284:errorcluster, "FP.State"=w282:T1)
            n114 = Not Equal?(x=w282, y=w280) -> (x != y?=w281:bool)
            n115 = case shown="True" w281 {
              tunnel: [w291 w292] -> w287
              tunnel: w284 -> [w290 w292]
              tunnel: w283 -> [w289 _]
              tunnel: w280 -> [w288 _]
              frame True {
                n116 = invoke class="VI" method="FP.Open"(reference=w289, error in=w290, "State"=w288) -> (error out=w291:errorcluster)  [unwired: 2 in, 4 out]
              }
              frame False {
              }
            }
          }
        }
        n117 = call <vilib>:"Add State(s) to Queue__JKI_lib_State_Machine.vi"("State(s) in (\"\")"=w227) -> ("States Out"=w226:string)  [unwired: 14 in]
      }
      frame "UI: LoadTabbedControls" {
        # "Initialize the User Interface, here.\n(this is called automatically, by the Macro: Init)"
        n118 = Unbundle By Name(w295) -> ("Core.Current VI Reference"=w299:refnum<vi>)
        n119 = control-ref of="Controls"() -> (w297:refnum<vi>)
        n120 = call "LoadTabbedControls.vi"("VI in"=w299) -> ("error out"=w296:errorcluster, "TabbedControls"=w298:T6[])  [unwired: 9 in]
        n121 = Bundle By Name(cluster=w295, "TabbedControls"=w298) -> (w300:T3)
        n122 = property class="MCListbox (strict)"(reference=w297, "SelColor"=u32 13816530, "Value"=-1) -> ()  [unwired: 1 in, 2 out]
        n123 = call <vilib>:"Add State(s) to Queue__JKI_lib_State_Machine.vi"("State(s) in (\"\")"=w302) -> ("States Out"=w301:string)  [unwired: 14 in]
      }
      frame "UI: VI Title String Update" {
        # "Do not put any code in this frame.\n(It is a separator no-op. You can make a copy of this frame to create a new UI frame)"
        n124 = Unbundle By Name(w312) -> ("Controls"=w303:T4[], "QuickDrop.VI Ref"=w305:refnum<vi>)
        n125 = property class="VI"(reference=w305) -> ("VIType"=w307:T7)  [unwired: 1 in, 2 out]
        n126 = Equal?(x=w307, y=T7."Control VI") -> (x = y?=w304:bool)
        n127 = case shown="False" w304 {
          tunnel: [w320 w321] -> w311
          tunnel: [w316 w322] -> w308
          tunnel: w305 -> [w315 _]
          tunnel: w303 -> [_ w325]
          frame False {
            n128 = property class="VI"(reference=w315) -> (error out=w320:errorcluster, "Front Panel.Title"=w318:string, "Front Panel.CustomTitle"=w319:bool, "Name"=w317:string)  [unwired: 1 in, 1 out]
            n129 = Select(t=w318, s=w319, f=w317) -> (s? t:f=w316:string)
          }
          frame True {
            n130 = Index Array(array=w325) -> (element=w324:T4)  [unwired: 1 in]
            n131 = Unbundle By Name(w324) -> ("Ref"=w323:refnum<vi>)
            n132 = property class="Ctl"(reference=w323) -> (error out=w321:errorcluster, "Label.Text"=w322:string)  [unwired: 1 in, 1 out]
          }
        }
        n133 = local write "VI Title"(w308) -> ()
        n134 = Merge Errors(w309, w311) -> (w310:errorcluster)
        n135 = call <vilib>:"Add State(s) to Queue__JKI_lib_State_Machine.vi"("State(s) in (\"\")"=w314) -> ("States Out"=w313:string)  [unwired: 14 in]
      }
      frame "UI: VI Description String Update" {
        # "Do not put any code in this frame.\n(It is a separator no-op. You can make a copy of this frame to create a new UI frame)"
        n136 = Unbundle By Name(w333) -> ("Controls"=w326:T4[], "QuickDrop.VI Ref"=w328:refnum<vi>)
        n137 = property class="VI"(reference=w328) -> ("VIType"=w330:T7)  [unwired: 1 in, 2 out]
        n138 = Equal?(x=w330, y=T7."Control VI") -> (x = y?=w327:bool)
        n139 = case shown="True" w327 {
          tunnel: [w338 w339] -> w332
          tunnel: [w337 w341] -> w331
          tunnel: w328 -> [w336 _]
          tunnel: w326 -> [_ w343]
          frame False {
            n140 = property class="VI"(reference=w336) -> (error out=w337:errorcluster, "Description"=w338:string)  [unwired: 1 in, 1 out]
          }
          frame True {
            n141 = Index Array(array=w343) -> (element=w342:T4)  [unwired: 1 in]
            n142 = Unbundle By Name(w342) -> ("Ref"=w340:refnum<vi>)
            n143 = property class="Ctl"(reference=w340) -> (error out=w341:errorcluster, "Desc"=w339:string)  [unwired: 1 in, 1 out]
          }
        }
        n144 = local write "Description"(w332) -> ()
        n145 = call <vilib>:"Add State(s) to Queue__JKI_lib_State_Machine.vi"("State(s) in (\"\")"=w335) -> ("States Out"=w334:string)  [unwired: 14 in]
      }
      frame "UI: Controls Update" {
        # "Do not put any code in this frame.\n(It is a separator no-op. You can make a copy of this frame to create a new UI frame)"
        n146 = Unbundle By Name(w352) -> ("Controls"=w345:T4[], "QuickDrop.VI Ref"=w349:refnum<vi>)
        n147 = property class="VI"(reference=w349) -> ("VIType"=w348:T7)  [unwired: 1 in, 2 out]
        n148 = Equal?(x=w348, y=T7."Standard VI") -> (x = y?=w346:bool)
        n149 = case shown="False" w346 {
          tunnel: w345 -> [w358 w359]
          tunnel: [w357 w359] -> w344
          frame False {
            n150 = Delete From Array(array=w358, length=1, index=0) -> (array with subset deleted=w357:T4[])  [unwired: 1 out]
          }
          frame True {
          }
        }
        n151 = control-ref of="ControlsListbox"() -> (w350:refnum<vi>)
        n152 = call "UpdateMCListboxFromControls.vi"("IncludeSymbols?"=w346, "Controls"=w344, "MulticolumnListbox in"=w350) -> ("error out"=w351:errorcluster)  [unwired: 8 in]
        n153 = call <vilib>:"Add State(s) to Queue__JKI_lib_State_Machine.vi"("State(s) in (\"\")"=w354) -> ("States Out"=w353:string)  [unwired: 14 in]
      }
      frame "---------- Macro ----------" {
        # "Do not put any code in this frame.\n(It is a separator no-op. You can make a copy of this frame to create a new Macro frame)"
        n154 = call <vilib>:"Add State(s) to Queue__JKI_lib_State_Machine.vi"("State(s) in (\"\")"=w363) -> ("States Out"=w362:string)  [unwired: 14 in]
      }
      frame "Macro: Initialize" {
        # "Initialization Macro\n(This is called once, when the VI starts)"
        n155 = call <vilib>:"Add State(s) to Queue__JKI_lib_State_Machine.vi"("State(s) in Front (\"\")"="Data: Initialize\nInitialize Core Data\n\nData: LoadControlFromVI\n\nUI: Initialize\nUI: LoadTabbedControls\n\nUI: VI Title String Update\nUI: VI Description String Update\nUI: Controls Update\n\nUI: Front Panel State >> Open", "State(s) in (\"\")"=w368) -> ("States Out"=w367:string)  [unwired: 13 in]
      }
      frame "Macro: Exit" {
        # "Remove KeyFocus to update\nlast input"
        # "Exit Macro\n(This is called once, when the VI exits)"
        n156 = Unbundle By Name(w377) -> ("Core.Close Panel on Exit?"=w376:bool)
        n157 = control-ref of="Help"() -> (w369:refnum<vi>)
        n158 = property class="Bool (strict)"(reference=w369, "Key Focus"=TRUE) -> ()  [unwired: 1 in, 2 out]
        n159 = Select(t="UI: Front Panel State >> Close", s=w376, f="") -> (s? t:f=w373:string)
        n160 = call <vilib>:"Add State(s) to Queue__JKI_lib_State_Machine.vi"("State(s) in (\"\")"=w373, "State(s) at Back (\"\")"="PropsUpdate: ViTitle\nPropsUpdate: ViDescription\nPropsUpdate: Controls\n\nData: Cleanup\nExit") -> ("States Out"=w371:string)  [unwired: 13 in]
        n161 = call <vilib>:"Add State(s) to Queue__JKI_lib_State_Machine.vi"("State(s) in Front (\"\")"=w371, "State(s) in (\"\")"=w380) -> ("States Out"=w379:string)  [unwired: 13 in]
      }
      frame "---------- PropsUpdate ----------" {
        # "Template Separator\n(You can make a copy of, or modify, this frame)"
        n162 = call <vilib>:"Add State(s) to Queue__JKI_lib_State_Machine.vi"("State(s) in (\"\")"=w384) -> ("States Out"=w383:string)  [unwired: 14 in]
      }
      frame "PropsUpdate: Reset ViTitle" {
        # "Reset VI Title to the VI name"
        n163 = Unbundle By Name(w391) -> ("QuickDrop.VI Ref"=w385:refnum<vi>)
        n164 = property class="VI"(reference=w385) -> ("VIType"=w387:T7)  [unwired: 1 in, 2 out]
        n165 = Equal?(x=w387, y=T7."Control VI") -> ()  [unwired: 1 out]
        n166 = property class="VI"(reference=w385) -> (error out=w390:errorcluster, "Name"=w392:string)  [unwired: 1 in, 1 out]
        n167 = local write "VI Title"(w392) -> ()
        n168 = Merge Errors(w388, w390) -> (w389:errorcluster)
        n169 = call <vilib>:"Add State(s) to Queue__JKI_lib_State_Machine.vi"("State(s) in (\"\")"=w394) -> ("States Out"=w393:string)  [unwired: 14 in]
      }
      frame "PropsUpdate: ViTitle" {
        # "Update the Frontpanel's Title"
        n170 = Unbundle By Name(w404) -> ("Controls"=w397:T4[], "QuickDrop.VI Ref"=w399:refnum<vi>)
        n171 = local read "VI Title"() -> (w402:string)
        n172 = property class="VI"(reference=w399) -> ("VIType"=w401:T7)  [unwired: 1 in, 2 out]
        n173 = Equal?(x=w401, y=T7."Control VI") -> (x = y?=w398:bool)
        n174 = case shown="True" w398 {
          tunnel: [w417 w421] -> w403
          tunnel: w402 -> [w408 w422]
          tunnel: w399 -> [w409 _]
          tunnel: w397 -> [_ w427]
          frame False {
            n175 = property class="VI"(reference=w409) -> (reference out=w412:refnum<vi>, "Front Panel.Title"=w411:string)  [unwired: 1 in, 1 out]
            n176 = Not Equal?(x=w411, y=w408) -> (x != y?=w410:bool)
            n177 = case shown="True" w410 {
              tunnel: [_ w420] -> w407
              tunnel: w408 -> [_ w419]
              tunnel: w412 -> [_ w418]
              frame False {
              }
              frame True {
                n178 = property class="VI"(reference=w418, "Front Panel.Title"=w419) -> (error out=w420:errorcluster)  [unwired: 1 in, 1 out]
              }
            }
            n179 = property class="VI"(reference=w409, error in=w407) -> (reference out=w416:refnum<vi>, error out=w413:errorcluster, "Name"=w415:string)
            n180 = Not Equal?(x=w415, y=w408) -> (x != y?=w414:bool)
            n181 = property class="VI"(reference=w416, error in=w413, "Front Panel.CustomTitle"=w414) -> (error out=w417:errorcluster)  [unwired: 1 out]
          }
          frame True {
            n182 = Index Array(array=w427, index=0) -> (element=w428:T4)
            n183 = Unbundle By Name(w428) -> ("Ref"=w423:refnum<vi>)
            n184 = property class="Ctl"(reference=w423) -> (reference out=w426:refnum<vi>, "Label.Text"=w425:string)  [unwired: 1 in, 1 out]
            n185 = Not Equal?(x=w425, y=w422) -> (x != y?=w424:bool)
            n186 = case shown="True" w424 {
              tunnel: [_ w432] -> w421
              tunnel: w422 -> [_ w431]
              tunnel: w426 -> [_ w430]
              frame False {
              }
              frame True {
                n187 = property class="Ctl"(reference=w430, "Label.Text"=w431) -> (error out=w432:errorcluster)  [unwired: 1 in, 1 out]
              }
            }
          }
        }
        n188 = Merge Errors(w395, w403) -> (w396:errorcluster)
        n189 = call <vilib>:"Add State(s) to Queue__JKI_lib_State_Machine.vi"("State(s) in (\"\")"=w406) -> ("States Out"=w405:string)  [unwired: 14 in]
      }
      frame "PropsUpdate: ViDescription" {
        # "Update description of the VI"
        n190 = Unbundle By Name(w442) -> ("Controls"=w435:T4[], "QuickDrop.VI Ref"=w437:refnum<vi>)
        n191 = local read "Description"() -> (w441:string)
        n192 = property class="VI"(reference=w437) -> ("VIType"=w439:T7)  [unwired: 1 in, 2 out]
        n193 = Equal?(x=w439, y=T7."Control VI") -> (x = y?=w436:bool)
        n194 = case shown="True" w436 {
          tunnel: w441 -> [w446 w454]
          tunnel: [w445 w459] -> w440
          tunnel: w437 -> [w447 _]
          tunnel: w435 -> [_ w462]
          frame False {
            n195 = property class="VI"(reference=w447) -> (reference out=w450:refnum<vi>, "Description"=w449:string)  [unwired: 1 in, 1 out]
            n196 = Not Equal?(x=w449, y=w446) -> (x != y?=w448:bool)
            n197 = case shown="True" w448 {
              tunnel: [_ w453] -> w445
              tunnel: w446 -> [_ w452]
              tunnel: w450 -> [_ w451]
              frame False {
              }
              frame True {
                n198 = property class="VI"(reference=w451, "Description"=w452) -> (error out=w453:errorcluster)  [unwired: 1 in, 1 out]
              }
            }
          }
          frame True {
            n199 = Index Array(array=w462, index=0) -> (element=w460:T4)
            n200 = Unbundle By Name(w460) -> ("Ref"=w458:refnum<vi>)
            n201 = property class="Ctl"(reference=w458) -> (reference out=w457:refnum<vi>, "Desc"=w456:string)  [unwired: 1 in, 1 out]
            n202 = Not Equal?(x=w456, y=w454) -> (x != y?=w455:bool)
            n203 = case shown="True" w455 {
              tunnel: [_ w465] -> w459
              tunnel: w454 -> [_ w464]
              tunnel: w457 -> [_ w463]
              frame False {
              }
              frame True {
                n204 = property class="Ctl"(reference=w463, "Desc"=w464) -> (error out=w465:errorcluster)  [unwired: 1 in, 1 out]
              }
            }
          }
        }
        n205 = Merge Errors(w433, w440) -> (w434:errorcluster)
        n206 = call <vilib>:"Add State(s) to Queue__JKI_lib_State_Machine.vi"("State(s) in (\"\")"=w444) -> ("States Out"=w443:string)  [unwired: 14 in]
      }
      frame "PropsUpdate: Controls" {
        # "Property Update of Control elements\n(You can make a copy of, or modify, this frame)"
        n207 = Unbundle By Name(w476) -> ("Controls"=w468:T4[], "QuickDrop.VI Ref"=w469:refnum<vi>)
        n208 = property class="VI"(reference=w469) -> ("VIType"=w471:T7)  [unwired: 1 in, 2 out]
        n209 = Equal?(x=w471, y=T7."Control VI") -> (x = y?=w466:bool)
        n210 = case shown="True" w466 {
          tunnel: w468 -> [w479 w481]
          tunnel: [w479 w480] -> w467
          frame False {
          }
          frame True {
            n211 = Delete From Array(array=w481, length=1, index=0) -> (array with subset deleted=w480:T4[])  [unwired: 1 out]
          }
        }
        n212 = control-ref of="Controls"() -> (w474:refnum<vi>)
        n213 = call "UpdateControlsFromMCListbox.vi"("MulticolumnListbox in"=w474, "Controls in"=w467) -> ("error out"=w475:errorcluster)  [unwired: 9 in]
        n214 = Merge Errors(w472, w475) -> (w473:errorcluster)
        n215 = call <vilib>:"Add State(s) to Queue__JKI_lib_State_Machine.vi"("State(s) in (\"\")"=w478) -> ("States Out"=w477:string)  [unwired: 14 in]
      }
    }
  }
  "error out" <- w1
